vi "FlyWheelSim_New.vi"(8 "MeasurementStdDev":T1, 9 "jKgMetersSquared":dbl, 10 "Gearing":dbl=1.0, 11 "GearBox":T2 {"Kt_NMPerAmp" format="%13.5p"; "Kv_RadPerSecPerVolt" format="%13.5p"; "R_Ohms" format="%13.5p"; "FreeSpeed_RadPerSec" format="%13.5p"; "FreeCurrent_Amps" format="%13.5p"; "StallCurrent_Amps" format="%13.5p"; "StallTorque_NM" format="%13.5p"; "nominalVoltage_Volts" format="%13.5p"}) -> (3 "FlyWheelSim":T3 {"GearBox"."Kt_NMPerAmp" format="%13.5p"; "GearBox"."Kv_RadPerSecPerVolt" format="%13.5p"; "GearBox"."R_Ohms" format="%13.5p"; "GearBox"."FreeSpeed_RadPerSec" format="%13.5p"; "GearBox"."FreeCurrent_Amps" format="%13.5p"; "GearBox"."StallCurrent_Amps" format="%13.5p"; "GearBox"."StallTorque_NM" format="%13.5p"; "GearBox"."nominalVoltage_Volts" format="%13.5p"})   [LabVIEW 2019, in "Trajectory_Library.lvlib"]
doc: "Creates a new LINEAR SYSTEM data cluster with the specified values. \n\n\nInputs: \n - XXX -- XXX.\n\nOutputs:\n - XXX -- XXX."
uses:
  Trajectory_Library.lvlib
  <vilib>/Analysis/Matrix/Datatypes/RealMatrix.ctl
  <vilib>/Analysis/Matrix/NI_Matrix.lvlib
  LINEAR_SYSTEM.ctl
  DCMOTOR.CTL
  FLYWHEEL_SIM.ctl
  LINEAR_SYSTEM_SIM.ctl
panel:
  # "<1, 1>"
  # "<States, 1>"
  # "<Outputs, 1>"
  # "<Inputs, 1>"
  # "<Outputs, 1>"
  # "<States,States>"
  # "<States,Inputs>"
  # "<Outputs,States>"
  # "<Outputs,Inputs>"
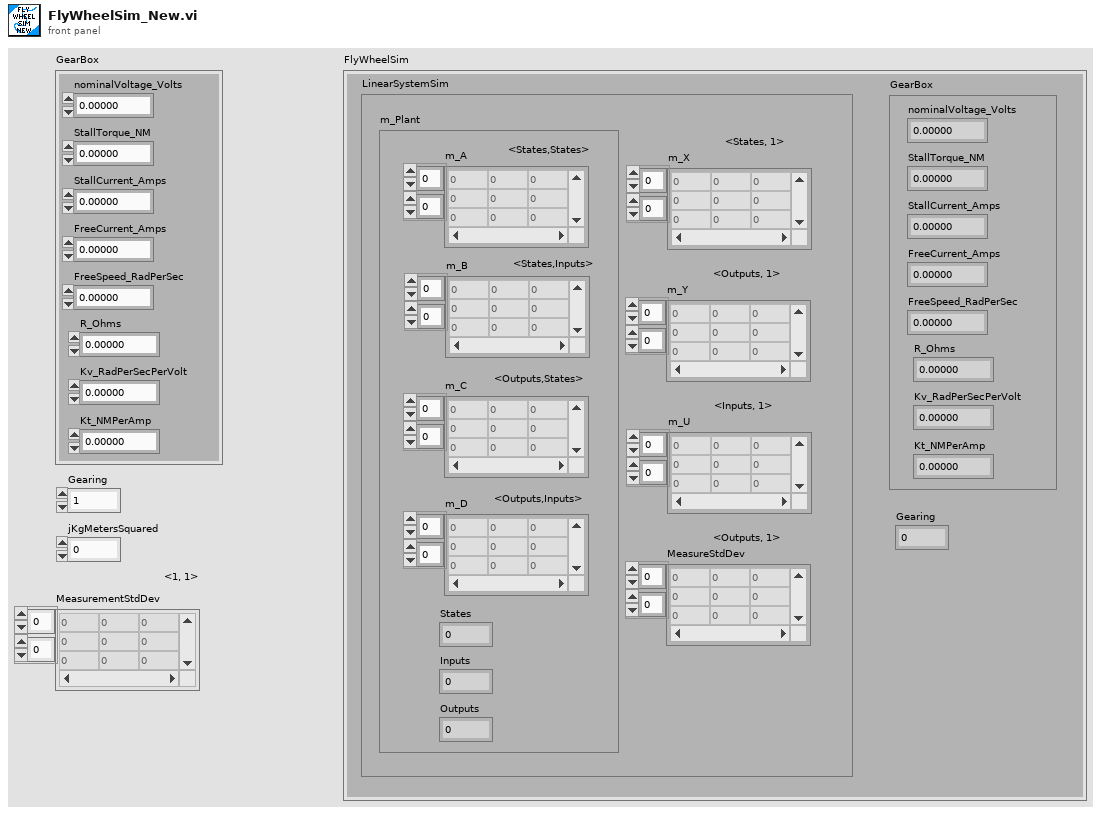
[diagram p1: front panel]
types:
  T1 = typedef "NI_Matrix.lvlib/RealMatrix.ctl" = dbl[][]
  T2 = typedef "Trajectory_Library.lvlib/DCMOTOR.CTL" = cluster{"nominalVoltage_Volts":dbl, "StallTorque_NM":dbl, "StallCurrent_Amps":dbl, "FreeCurrent_Amps":dbl, "FreeSpeed_RadPerSec":dbl, "R_Ohms":dbl, "Kv_RadPerSecPerVolt":dbl, "Kt_NMPerAmp":dbl}
  T3 = typedef "Trajectory_Library.lvlib/FLYWHEEL_SIM.ctl" = cluster{"LinearSystemSim":T4, "GearBox":T2, "Gearing":dbl}
  T4 = typedef "Trajectory_Library.lvlib/LINEAR_SYSTEM_SIM.ctl" = cluster{"m_Plant":T5, "m_X":T1, "m_Y":T1, "m_U":T1, "MeasureStdDev":T1}
  T5 = typedef "Trajectory_Library.lvlib/LINEAR_SYSTEM.ctl" = cluster{"m_A":T1, "m_B":T1, "m_C":T1, "m_D":T1, "States":i32, "Inputs":i32, "Outputs":i32}
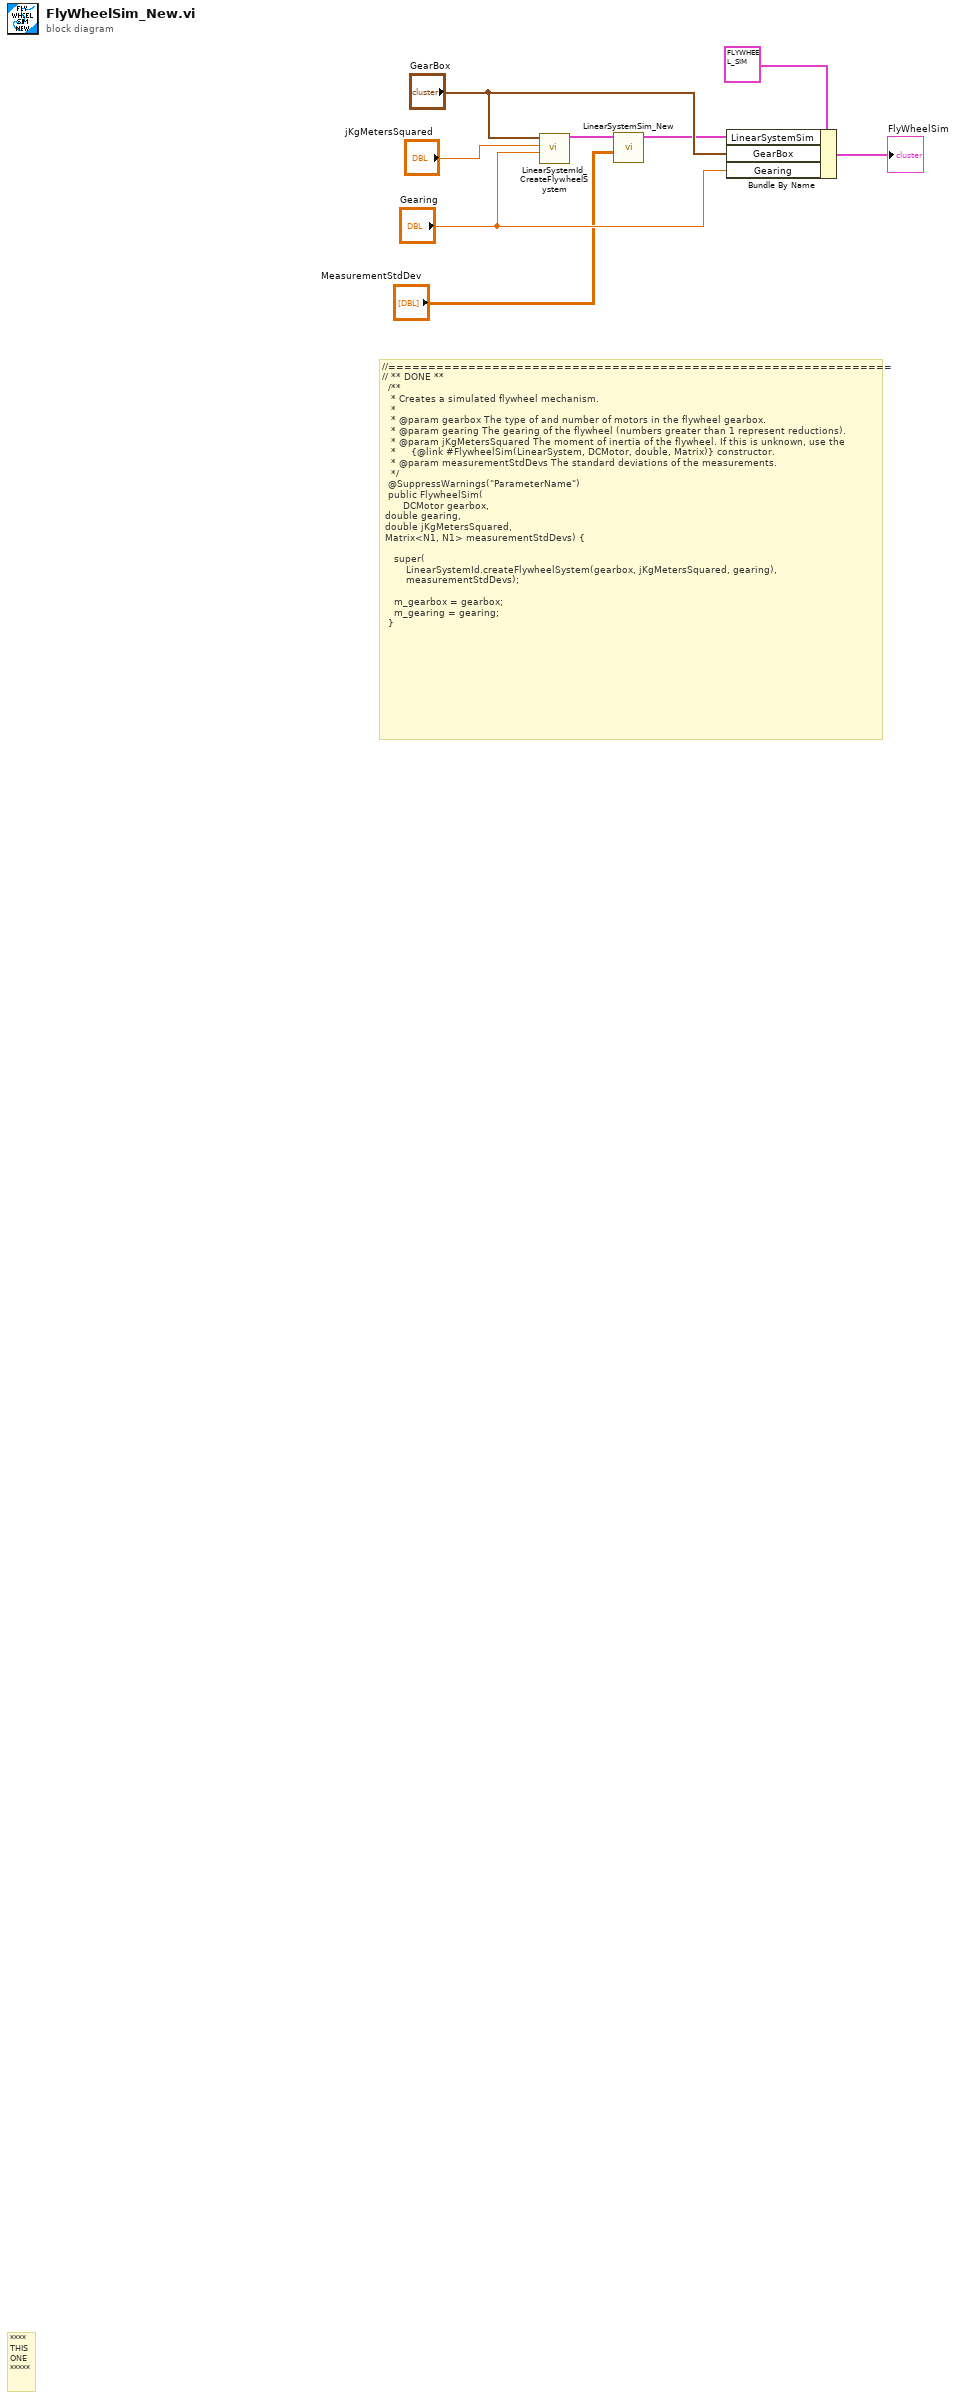
[diagram p0: block diagram]
diagram:
  # "//===============================================================\n// ** DONE **\n  /**\n   * Creates a simulated flywheel mechanism.\n   *\n   * @param gearbox The type of and number of motors in the flywheel gearbox.\n   * @param gearing The gearing of the flywheel (numbers greater than 1 represent reductions).\n   * @param jKgMetersSquared The moment of inertia of the flywheel. If this is unknown, use the\n   *     {@link #FlywheelSim(LinearSystem, DCMotor, double, Matrix)} constructor.\n   * @param measurementStdDevs The standard deviations of the measurements.\n   */\n  @SuppressWarnings(\"ParameterName\")\n  public FlywheelSim(\n      \tDCMotor gearbox, \n\tdouble gearing, \n\tdouble jKgMetersSquared, \n\tMatrix<N1, N1> measurementStdDevs) {\n\n    super(\n        LinearSystemId.createFlywheelSystem(gearbox, jKgMetersSquared, gearing),\n        measurementStdDevs);\n\n    m_gearbox = gearbox;\n    m_gearing = gearing;\n  }"
  # "****\nTHIS\nONE\n*****"
  n1 = call "LinearSystemId_CreateFlywheelSystem.vi"("G"="Gearing", "jKgMetersSquared"="jKgMetersSquared", "DCMOTOR"="GearBox") -> ("Linearsystem"=w3:T5)  [unwired: 8 in]
  n2 = call "LinearSystemSim_New.vi"("MeasurementStdDev"="MeasurementStdDev", "System"=w3) -> ("LinearSystemSim"=w1:T4)  [unwired: 9 in]
  n3 = Bundle By Name(cluster=T3 {"LinearSystemSim"={"m_Plant"={"m_A"=[], "m_B"=[], "m_C"=[], "m_D"=[], "States"=0, "Inputs"=0, "Outputs"=0}, "m_X"=[], "m_Y"=[], "m_U"=[], "MeasureStdDev"=[]}, "GearBox"={"nominalVoltage_Volts"=0.0, "StallTorque_NM"=0.0, "StallCurrent_Amps"=0.0, "FreeCurrent_Amps"=0.0, "FreeSpeed_RadPerSec"=0.0, "R_Ohms"=0.0, "Kv_RadPerSecPerVolt"=0.0, "Kt_NMPerAmp"=0.0}, "Gearing"=0.0} ("FLYWHEEL_SIM"), "LinearSystemSim"=w1, "GearBox"="GearBox", "Gearing"="Gearing") -> (→"FlyWheelSim":T3)
